vi "Multiple_File_Opener_Tester.vi"() -> ()   [LabVIEW 2023]
uses:
  <vilib>/Utility/file.llb/Read Delimited Spreadsheet (string).vi
  <vilib>/Utility/file.llb/Read Delimited Spreadsheet (DBL).vi
panel:
  in  "stop":bool
  in  "EEG Signals":path
  out "Header of EEGs":string[](array[string])
  out "Dataset of EEGs":dbl[][](array[numeric])
  out "appended path":path
  in  "Base Folder":path=path "C:/Users/AIIH/Documents/LabVIEW/EEG/Filtered_Data"
  in  "Boolean":bool
  in  "Files":path=path "C:/Users/AIIH/Documents/LabVIEW/EEG/RECORDS_1.csv"
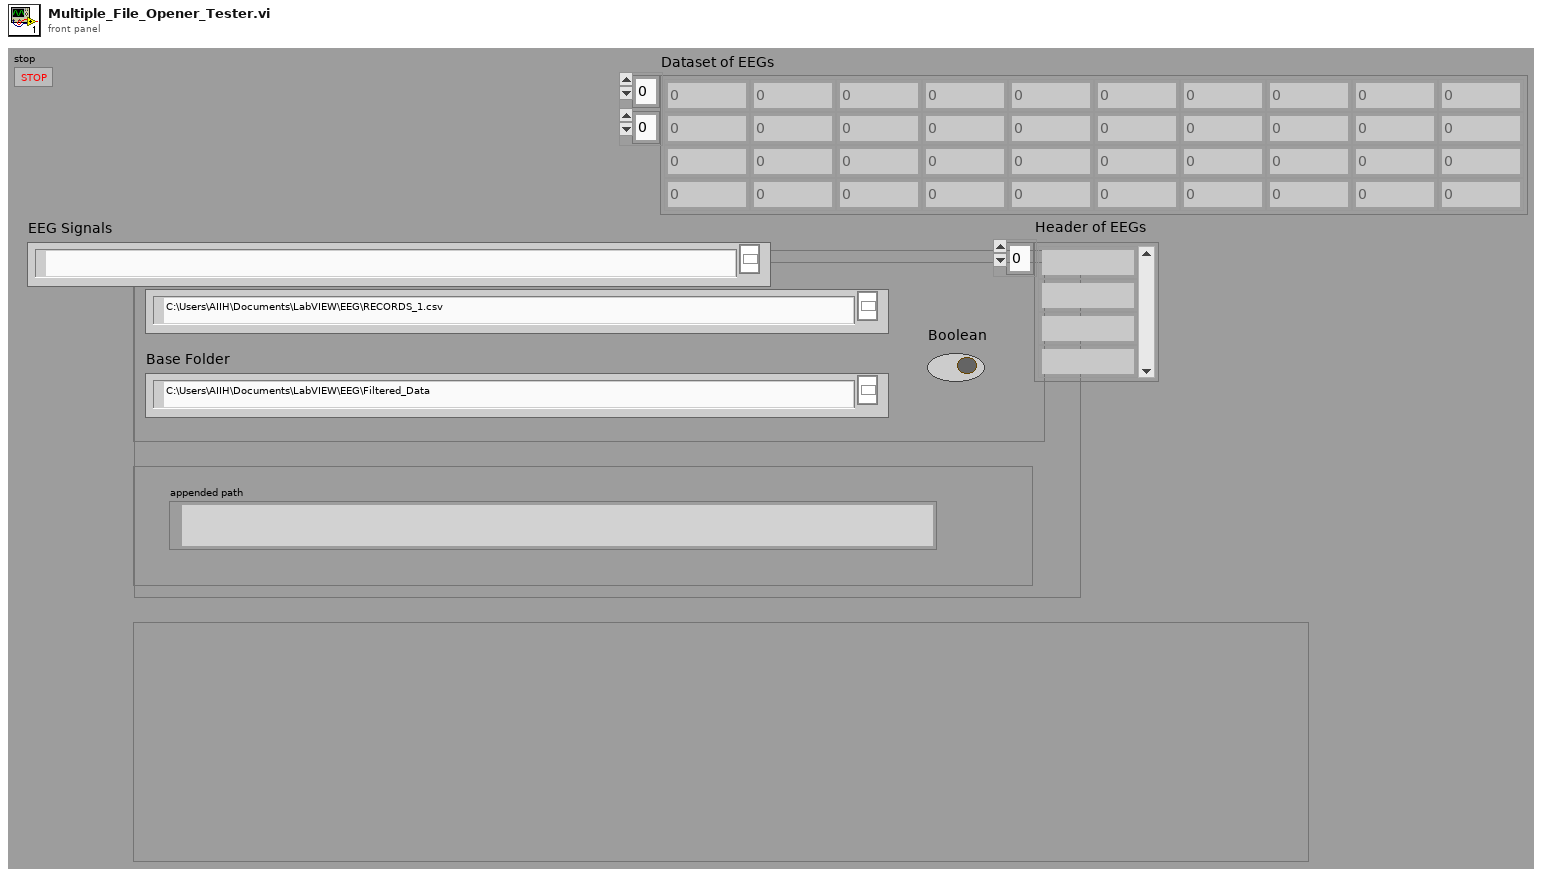
[diagram p1: front panel]
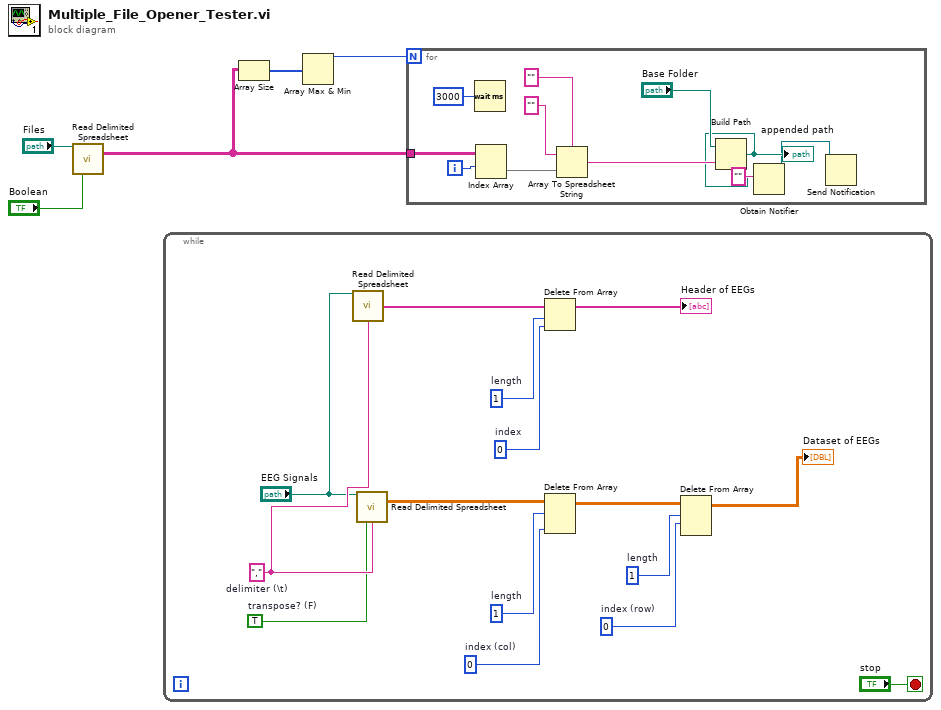
[diagram p0: block diagram]
diagram:
  n1 = call-poly <vilib>:"Read Delimited Spreadsheet.vi"("file path (dialog if empty)"="Files", "transpose? (F)"="Boolean") -> ("all rows"=w3:string[][])  [unwired: 8 in, 5 out]
  n2 = while {
    stop <- "stop" stop-if-true
    w9 = TRUE  # transpose? (F)
    w10 = 0  # index
    w11 = 1  # length
    w14 = 0  # index (row)
    w15 = 1  # length
    w17 = 0  # index (col)
    w18 = 1  # length
    w20 = ","  # delimiter (\t)
    n3 = call-poly <vilib>:"Read Delimited Spreadsheet.vi"("file path (dialog if empty)"="EEG Signals", "delimiter (\\t)"=w20) -> ("first row"=w13:string[])  [unwired: 8 in, 5 out]
    n4 = call-poly <vilib>:"Read Delimited Spreadsheet.vi"("file path (dialog if empty)"="EEG Signals", "transpose? (F)"=w9, "delimiter (\\t)"=w20) -> ("all rows"=w19:dbl[][])  [unwired: 7 in, 5 out]
    n5 = Delete From Array "Delete From Array"(array=w13, length=w11, index=w10) -> (array with subset deleted=→"Header of EEGs":string[])  [unwired: 1 out]
    n6 = Delete From Array "Delete From Array"(array=w19, length=w18, index (col)=w17) -> (array with subset deleted=w16:dbl[][])  [unwired: 1 in, 1 out]
    n7 = Delete From Array "Delete From Array"(array=w16, length=w15, index (row)=w14) -> (array with subset deleted=→"Dataset of EEGs":dbl[][])  [unwired: 1 in, 1 out]
  }
  n8 = Array Size(array=w3) -> (size(s)=w2:i32[])
  n9 = Array Max & Min(array=w2) -> (max value=w1:i32)  [unwired: 3 out]
  n10 = for {
    N: w1 -> [_]
    tunnel: w3 -> [w31]
    i -> [w30]
    n11 = Wait (ms)(milliseconds to wait=u32 3000) -> ()  [unwired: 1 out]
    n12 = Index Array "Index Array"(array=w31, index (row)=w30) -> (element=w27:string[])  [unwired: 1 in]
    n13 = Array To Spreadsheet String(delimiter (Tab)="", array=w27, 3:"" ("format string")) -> (spreadsheet string=w28:string)
    n14 = Build Path(base path="Base Folder", name or relative path=w28) -> (appended path=w22:path)
    "appended path" <- w22
    n15 = Obtain Notifier(name (unnamed)="", notification data type=w22) -> (notifier out=w21:refnum<notifier>)  [unwired: 2 in, 2 out]
    n16 = Send Notification(notifier=w21) -> ()  [unwired: 2 in, 2 out]
  }
